vi "DropVI_SimpleClient_Pub-Sub.vi"() -> ()   [LabVIEW 2013, in "MQTT Client.lvlib"]
uses:
  MQTT Client.lvlib
  <vilib>/LabVIEW Open Source Project/MQTT Connection/MQTT_Connection/Connection/Connection.lvclass
  Client class/Client.lvclass/Client.ctl
  <vilib>/LabVIEW Open Source Project/MQTT Connection/MQTT_Base/Base Class/MQTT_Base.lvclass/MQTT_Base.ctl
  <vilib>/LabVIEW Open Source Project/MQTT Control Packets/Control Packets/ControlPacket/QualityOfService -- enum.ctl
  <vilib>/LabVIEW Open Source Project/MQTT Control Packets/Control Packets/CONNECT/ConnectFlags -- cluster.ctl
  <vilib>/LabVIEW Open Source Project/MQTT Control Packets/Control Packets/PUBLISH/PUBLISH.lvclass
  Client class/Client.lvclass
  <vilib>/LabVIEW Open Source Project/MQTT Connection/MQTT_Base/Base Class/MQTT_Base.lvclass
  <vilib>/LabVIEW Open Source Project/MQTT Control Packets/Control Packets/CONNECT/CONNECT.lvclass
  <vilib>/LabVIEW Open Source Project/MQTT Control Packets/Control Packets/ControlPacket/ControlPacket.lvclass
panel:
  out "Published":bool
  out "last error":errorcluster
  out "Unsuback":bool
  in  "Subscribe":bool
  in  "Connection":bool
  out "Waveform Chart":dbl(graph)
  out "Suback":bool
  in  "Stop Client":bool
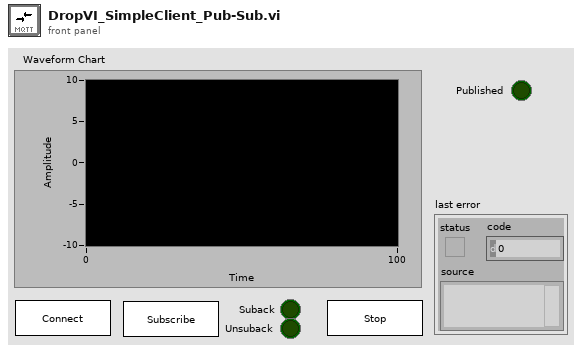
[diagram p1: front panel]
types:
  T1 = typedef "MQTT Client.lvlib/Client.lvclass/Public Events -- cluster.ctl" = cluster{"Connection Status":refnum<user-event>, "Connected":refnum<user-event>, "Application Message":refnum<user-event>}
  T2 = typedef "MQTT Base.lvlib/MQTT_Base.lvclass/Public Events -- cluster.ctl" = cluster{"Stop Event":refnum<user-event>, "Error Event":refnum<user-event>, "Inbound Message":refnum<user-event>}
  T3 = typedef "MQTT_Control_Packets.lvlib/ControlPacket.lvclass/QualityOfService -- enum.ctl" = enum16{"0 (At Most Once)", "1 (At Least Once)", "2 (Exactly Once)"}
  T4 = typedef "MQTT_Control_Packets.lvlib/CONNECT.lvclass/ConnectFlags -- cluster.ctl" = cluster{"Reserved":bool, "Clean Session":bool, "Will Flag":bool, "Will QoS 1":bool, "Will QoS 2":bool, "Will Retain":bool, "Password Flag":bool, "User Name Flag":bool}
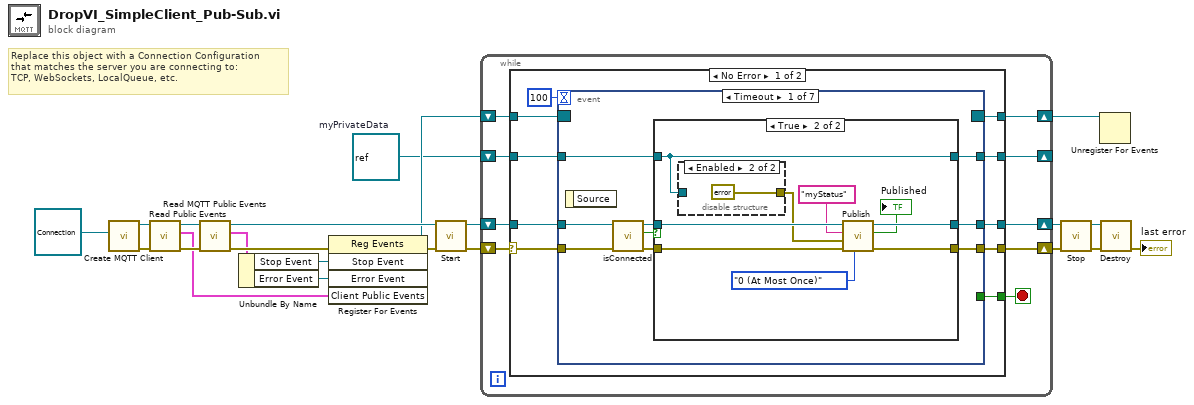
[diagram p0: block diagram]
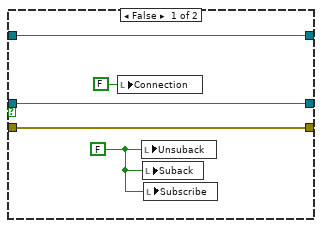
[diagram p2: hidden frame]
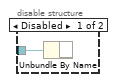
[diagram p3: hidden frame]
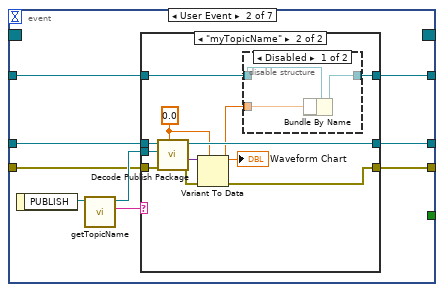
[diagram p4: hidden frame]
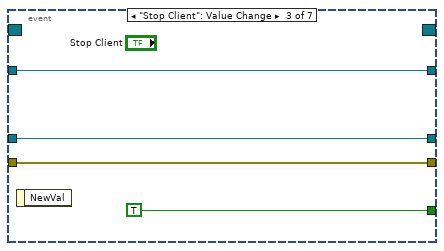
[diagram p7: hidden frame]
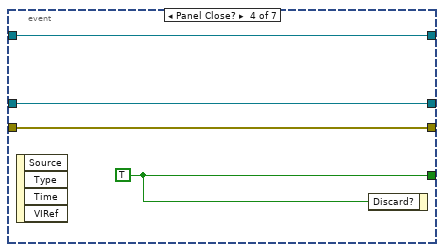
[diagram p8: hidden frame]
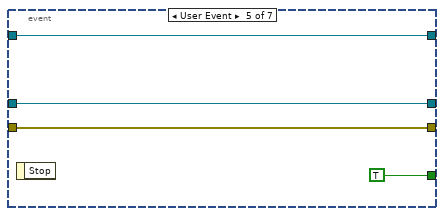
[diagram p9: hidden frame]
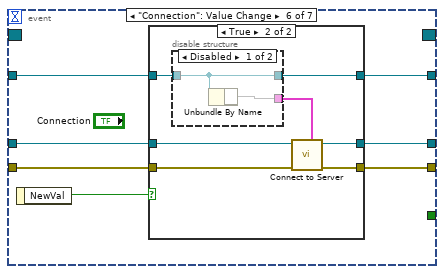
[diagram p10: hidden frame]
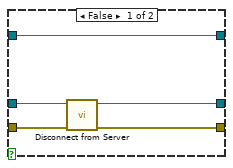
[diagram p11: hidden frame]
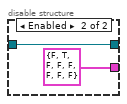
[diagram p12: hidden frame]
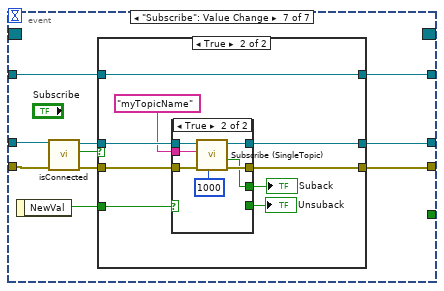
[diagram p13: hidden frame]
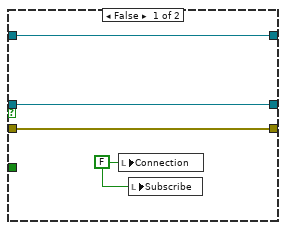
[diagram p14: hidden frame]
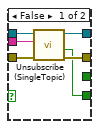
[diagram p15: hidden frame]
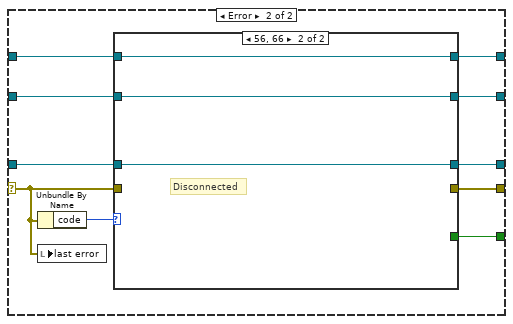
[diagram p16: hidden frame]
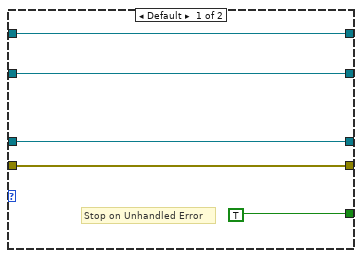
[diagram p17: hidden frame]
diagram:
  w1 = refnum<class> refnum  # myPrivateData
  # "Replace this object with a Connection Configuration\nthat matches the server you are connecting to:\nTCP, WebSockets, LocalQueue, etc."
  n1 = call "Create MQTT Client.vi"("Connection Configuration"=refnum<class "Connection.lvclass"> refnum) -> ("error out"=w20:errorcluster, "Client out"=w22:refnum<class "Client.lvclass">)  [unwired: 9 in]
  n2 = call "Read Public Events.vi"("error in (no error)"=w20, "Client in"=w22) -> ("error out"=w19:errorcluster, "Client Public Events"=w17:T1, "Client out"=w21:refnum<class "Client.lvclass">)  [unwired: 7 in]
  n3 = call <vilib>:"Read MQTT Public Events.vi"("error in (no error)"=w19, "MQTT_Base in"=w21) -> ("error out"=w18:errorcluster, "MQTT Public Events"=w10:T2, "MQTT_Base out"=w15:refnum<class "Client.lvclass">)  [unwired: 7 in]
  n4 = Unbundle By Name(w10) -> ("Stop Event"=w12:refnum<user-event>, "Error Event"=w11:refnum<user-event>)
  n5 = register-events(error in=w18, w12, w11, w17) -> (reference out=w14:refnum<event-registration>, error out=w16:errorcluster)  [unwired: 1 in]
  n6 = call <vilib>:"Start.vi"("error in (no error)"=w16, "MQTT_Base in"=w15) -> ("error out"=w3:errorcluster, "MQTT_Base out"=w4:refnum<class "Client.lvclass">)  [unwired: 7 in, 1 out]
  n7 = while {
    shift-right: [w30] -> w13
    shift-left: w14 -> [w31]
    shift-right: [w27] -> w7
    shift-left: w4 -> [w28]
    shift-right: [w29] -> w5
    shift-left: w3 -> [w25]
    shift-right: [w23] -> _
    shift-left: w1 -> [w24]
    stop <- w26 stop-if-true
    n8 = case shown="No Error" w25 {
      selector: w25 -> [w34 w168]
      tunnel: w31 -> [w41 w167]
      tunnel: [w40 w166] -> w30
      tunnel: [w39 w171] -> w29
      tunnel: w28 -> [w37 w172]
      tunnel: [w36 w174] -> w27
      tunnel: [w35 w170] -> w26
      tunnel: w24 -> [w33 w169]
      tunnel: [w32 w165] -> w23
      frame No Error {
        n9 = event shown="[0] Timeout" {
          selector: w41 -> [_ _ _ _ _ _ _]
          dyn-events: [_ _ _ _ _ _ _] -> w40
          timeout: 100 -> [_ _ _ _ _ _ _]
          tunnel: w34 -> [w46 w72 w96 w99 w105 w108 w136]
          tunnel: [w49 w69 w96 w99 w105 w109 w137] -> w39
          tunnel: [_ _ TRUE w101 TRUE _ _] -> w35
          tunnel: w37 -> [w48 w73 w97 w100 w103 w112 w135]
          tunnel: [w50 w71 w97 w100 w103 w110 w138] -> w36
          tunnel: w33 -> [w43 w68 w94 w98 w102 w106 w130]
          tunnel: [w42 w67 w94 w98 w102 w107 w129] -> w32
          event Timeout {
            n10 = event-data() -> ()  [unwired: 1 in, 1 out]
            n11 = call "isConnected.vi"("error in (no error)"=w46, "Client in"=w48) -> ("error out"=w45:errorcluster, "connected"=w44:bool, "Client out"=w47:refnum<class "Client.lvclass">)  [unwired: 7 in]
            n12 = case shown="True" w44 {
              tunnel: [w55 w63] -> w50
              tunnel: [w54 w61] -> w49
              tunnel: w47 -> [w55 w64]
              tunnel: w45 -> [w54 w62]
              tunnel: w43 -> [w51 w59]
              tunnel: [w51 w59] -> w42
              frame False {
                w53 = FALSE
                n13 = local write "Connection"(FALSE ("Connection")) -> ()
                n14 = local write "Unsuback"(w53) -> ()
                n15 = local write "Suback"(w53) -> ()
                n16 = local write "Subscribe"(w53) -> ()
              }
              frame True {
                n17 = disable-structure shown="Enabled" {
                  disable-tunnel: w59 -> [w65 _]
                  disable-tunnel: [_ errorcluster {"status"=FALSE, "code"=0, "source"=""} ("error constant")] -> w58
                  frame Disabled {
                    n18 = Unbundle By Name(w65) -> ()  [unwired: 1 out]
                  }
                  frame Enabled {
                  }
                }
                n19 = call "Publish.vi"("QoS"=QualityOfService_--_enum."0 (At Most Once)", "error in (no error)"=w62, "Payload"=w58, "Topic Name (empty: Payload name)"="myStatus", "Client in"=w64) -> ("error out"=w61:errorcluster, "Published"=→"Published":bool, "Client out"=w63:refnum<class "Client.lvclass">)  [unwired: 4 in]
              }
            }
          }
          event User Event {
            n20 = event-data() -> ("PUBLISH"=w75:refnum<class "PUBLISH.lvclass">)  [unwired: 1 in]
            n21 = call <vilib>:"getTopicName.vi"("PUBLISH in"=w75) -> ("Topic"=w70:string, "PUBLISH out"=w74:refnum<class "PUBLISH.lvclass">)  [unwired: 8 in, 1 out]
            n22 = case shown="\"myTopicName\"" w70 {
              tunnel: w74 -> [_ w89]
              tunnel: w73 -> [w78 w88]
              tunnel: w72 -> [w77 w87]
              tunnel: [w78 w86] -> w71
              tunnel: [w77 w82] -> w69
              tunnel: w68 -> [w76 w81]
              tunnel: [w76 w80] -> w67
              frame Default {
              }
              frame "myTopicName" {
                w84 = 0.0
                n23 = call <vilib>:"Decode Publish Package.vi"("Type"=w84, "error in (no error)"=w87, "PUBLISH"=w89, "MQTT_Base in"=w88) -> ("error out"=w83:errorcluster, "Payload"=w85:variant, "MQTT_Base out"=w86:refnum<class "Client.lvclass">)  [unwired: 4 in, 1 out]
                n24 = Variant To Data(error in=w83, type=w84, Variant=w85) -> (data=w79:dbl, error out=w82:errorcluster)
                "Waveform Chart" <- w79
                n25 = disable-structure shown="Disabled" {
                  disable-tunnel: w81 -> [w90 w93]
                  disable-tunnel: [w92 w93] -> w80
                  disable-tunnel: w79 -> [w91 _]
                  frame Disabled {
                    n26 = Bundle By Name(cluster=w90, w91) -> (w92:refnum<class>)
                  }
                  frame Enabled {
                  }
                }
              }
            }
          }
          event "Stop Client": Value Change {
            n27 = event-data() -> ()  [unwired: 1 in, 1 out]
          }
          event Panel Close? {
            w101 = TRUE
            n28 = event-data() -> ()  [unwired: 1 in, 4 out]
            n29 = event-data("Discard?"=w101) -> ()  [unwired: 1 in, 1 out]
          }
          event User Event {
            n30 = event-data() -> ()  [unwired: 1 in, 1 out]
          }
          event "Connection": Value Change {
            n31 = event-data() -> ("NewVal"=w111:bool)  [unwired: 1 in]
            n32 = case shown="True" w111 {
              tunnel: w112 -> [w117 w124]
              tunnel: [w116 w121] -> w110
              tunnel: [w115 w122] -> w109
              tunnel: w108 -> [w114 w123]
              tunnel: [w113 w119] -> w107
              tunnel: w106 -> [w113 w120]
              frame False {
                n33 = call "Disconnect from Server.vi"("error in (no error)"=w114, "Client in"=w117) -> ("error out"=w115:errorcluster, "Client out"=w116:refnum<class "Client.lvclass">)  [unwired: 7 in, 1 out]
              }
              frame True {
                n34 = disable-structure shown="Disabled" {
                  disable-tunnel: w120 -> [w126 w128]
                  disable-tunnel: [w126 w128] -> w119
                  disable-tunnel: [w125 T4 {"Reserved"=FALSE, "Clean Session"=TRUE, "Will Flag"=FALSE, "Will QoS 1"=FALSE, "Will QoS 2"=FALSE, "Will Retain"=FALSE, "Password Flag"=FALSE, "User Name Flag"=FALSE} ("Connect Flags")] -> w118
                  frame Disabled {
                    n35 = Unbundle By Name(w126) -> (w125)
                  }
                  frame Enabled {
                  }
                }
                n36 = call "Connect to Server.vi"("Connect Flags"=w118, "error in (no error)"=w123, "Client in"=w124) -> ("error out"=w122:errorcluster, "Client out"=w121:refnum<class "Client.lvclass">)  [unwired: 5 in, 2 out]
              }
            }
          }
          event "Subscribe": Value Change {
            n37 = event-data() -> ("NewVal"=w131:bool)  [unwired: 1 in]
            n38 = call "isConnected.vi"("error in (no error)"=w136, "Client in"=w135) -> ("error out"=w133:errorcluster, "connected"=w132:bool, "Client out"=w134:refnum<class "Client.lvclass">)  [unwired: 7 in]
            n39 = case shown="True" w132 {
              tunnel: [w142 w151] -> w138
              tunnel: [w141 w150] -> w137
              tunnel: w134 -> [w142 w149]
              tunnel: w133 -> [w141 w148]
              tunnel: w131 -> [_ w146]
              tunnel: w130 -> [w139 w143]
              tunnel: [w139 w143] -> w129
              frame False {
                w140 = FALSE ("Connection")
                n40 = local write "Connection"(w140) -> ()
                n41 = local write "Subscribe"(w140) -> ()
              }
              frame True {
                n42 = case shown="True" w146 {
                  tunnel: [w153 w163] -> w151
                  tunnel: [w157 w162] -> w150
                  tunnel: w149 -> [w156 w161]
                  tunnel: w148 -> [w155 w160]
                  tunnel: "myTopicName" ("Topic Name (empty: Payload name)") -> [w154 w159]
                  tunnel: [_ w158] -> w145
                  tunnel: [w152 _] -> w144
                  frame False {
                    n43 = call <vilib>:"Unsubscribe (SingleTopic).vi"("error in (no error)"=w155, "Topic Filter"=w154, "MQTT_Base in"=w156) -> ("error out"=w157:errorcluster, "Ack"=w152:bool, "MQTT_Base out"=w153:refnum<class "Client.lvclass">)  [unwired: 6 in]
                  }
                  frame True {
                    n44 = call <vilib>:"Subscribe (SingleTopic).vi"("timeout (100ms)"=1000, "error in (no error)"=w160, "Topic Filter"=w159, "MQTT_Base in"=w161) -> ("error out"=w162:errorcluster, "Ack"=w158:bool, "MQTT_Base out"=w163:refnum<class "Client.lvclass">)  [unwired: 5 in]
                  }
                }
                "Unsuback" <- w144
                "Suback" <- w145
              }
            }
          }
        }
      }
      frame Error {
        n45 = Unbundle By Name(w168) -> ("code"=w173:i32)
        n46 = local write "last error"(w168) -> ()
        n47 = case shown="56, 66" w173 {
          tunnel: w172 -> [w179 w182]
          tunnel: [w179 w182] -> w174
          tunnel: w168 -> [w178 _]
          tunnel: [w178 _] -> w171
          tunnel: [TRUE _] -> w170
          tunnel: w169 -> [w175 w180]
          tunnel: w167 -> [w176 w181]
          tunnel: [w176 w181] -> w166
          tunnel: [w175 w180] -> w165
          frame Default {
            # "Stop on Unhandled Error"
          }
          frame 56, 66 {
            # "Disconnected"
          }
        }
      }
    }
  }
  n48 = call <vilib>:"Stop.vi"("error in (no error)"=w5, "MQTT_Base in"=w7) -> ("error out"=w6:errorcluster, "MQTT_Base out"=w8:refnum<class "Client.lvclass">)  [unwired: 7 in, 1 out]
  n49 = Unregister For Events(event registration refnum=w13) -> ()  [unwired: 1 in, 1 out]
  n50 = call <vilib>:"Destroy.vi"("error in (no error)"=w6, "MQTT_Base in"=w8) -> ("error out"=→"last error":errorcluster)  [unwired: 8 in, 1 out]
